vi "PicoScope6000UnitInfo.vi"(7 "Mode":u16(ring) items=["Dialog On Error", "no dialog - CloseUnit and Stop", "no dialog - Continue", "no dialog - Stop"], 8 "error in (no error)":errorcluster, 11 "handle in":i16) -> (0 "error out":errorcluster, 3 "handle out":i16, 4 "Unit Info":T1)   [LabVIEW 2009]
uses:
  ps6000.dll
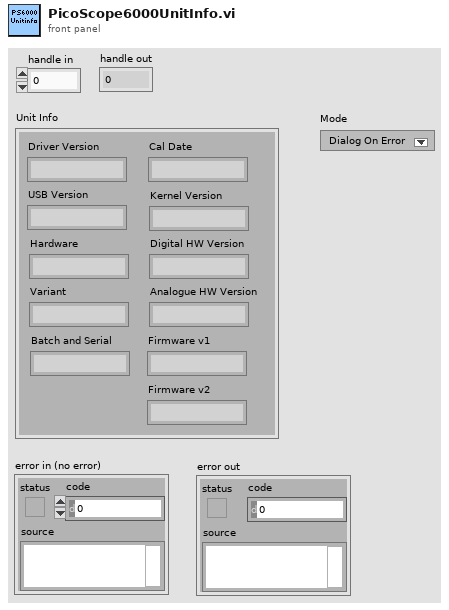
[diagram p1: front panel]
types:
  T1 = cluster{"Driver Version":string, "USB Version":string, "Hardware":string, "Variant":string, "Batch and Serial":string, "Cal Date":string, "Kernel Version":string, "Digital HW Version":string, "Analogue HW Version":string, "Firmware v1":string, "Firmware v2":string}
  T2 = cluster{"status":bool, "code":u32, "source":string}
  T3 = cluster{"[0]":string, "[1]":string, "[2]":string, "[3]":string, "[4]":string, "[5]":string, "[6]":string, "[7]":string, "[8]":string, "[9]":string, "[10]":string}
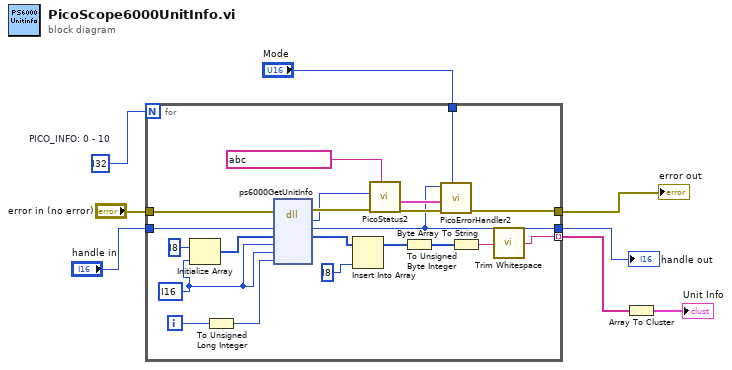
[diagram p0: block diagram]
diagram:
  w7 = i32 ?  # PICO_INFO: 0 - 10
  n1 = for {
    N: w7 -> [_]
    tunnel: "handle in" -> [w29]
    tunnel: [w11] -> w4 mode=indexing
    tunnel: "error in (no error)" -> [w28]
    tunnel: [w21] -> w5
    tunnel: [w24] -> w2
    tunnel: "Mode" -> [w13]
    i -> [w9]
    w20 = i16 ? ("stringLength")
    n2 = Initialize Array(i8 ? ("element"), w20) -> (w18:i8[])
    n3 = To Unsigned Long Integer(number=w9) -> (unsigned 32bit integer=w10:u32)
    n4 = dll-call lib="ps6000.dll" fn="ps6000GetUnitInfo"(error in=w28, "handle"=w29, "unitInfo"=w18, "stringLength"=w20, "requiredSize"=w20, "PICO_INFO"=w10) -> (error out=w25:errorcluster, "PICO_STATUS"=w23:u32, "handle"=w21:i16, "unitInfo"=w16:i8[])  [unwired: 5 in, 1 out]
    n5 = Insert Into Array(array=w16, new element=i8 ? ("new element/subarray")) -> (w14:i8[])  [unwired: 1 in]
    n6 = call "PicoStatus2.vi"("PICO source"=string ? ("source"), "Error in"=w25, "PICO STATUS"=w23) -> ("error out"=w27:errorcluster, "PICO_STATUS out"=w26:T2)  [unwired: 5 in]
    n7 = To Unsigned Byte Integer(number=w14) -> (unsigned 8bit integer=w15:u8[])
    n8 = call "PicoErrorHandler2.vi"("Mode"=w13, "error in (no error)"=w27, "PICO_STATUS in"=w26, "handle In"=w21) -> ("error out"=w24:errorcluster)  [unwired: 7 in]
    n9 = Byte Array To String(unsigned byte array=w15) -> (string=w12:string)
    n10 = call <vilib>:"Trim Whitespace.vi"("string"=w12) -> ("trimmed string"=w11:string)  [unwired: 1 in]
  }
  "error out" <- w2
  "handle out" <- w5
  n11 = Array To Cluster(array=w4) -> (cluster=→"Unit Info":T3)
